vi "ViconIMUSimulation.vi"() -> ()   [LabVIEW 2016]
uses:
  DataProcess/CAlex2-Data/CAlex2_Data.lvclass
  D:/JinXin/LabVIEW.git/CAlex2-Controller-treadmill/Sim&Process/DataProcess/ExpData/ExpData.lvclass
  Classes/CAlex2-Display/CAlex2_Display.lvclass
  D:/JinXin/LabVIEW.git/CAlex2-Controller-treadmill/Classes/SerialChain/SerialChain.lvclass
  Classes/CAlex2/CAlex2.lvclass
  DataProcess/ExpData/ExpData.lvclass
  Classes/SerialChain/SerialChain.lvclass
panel:
  in  "New":refnum<k7>(container)
  in  "Old":refnum<k7>(container)
  in  "Path":path
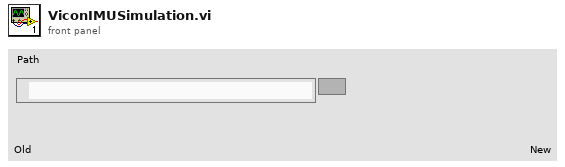
[diagram p1: front panel]
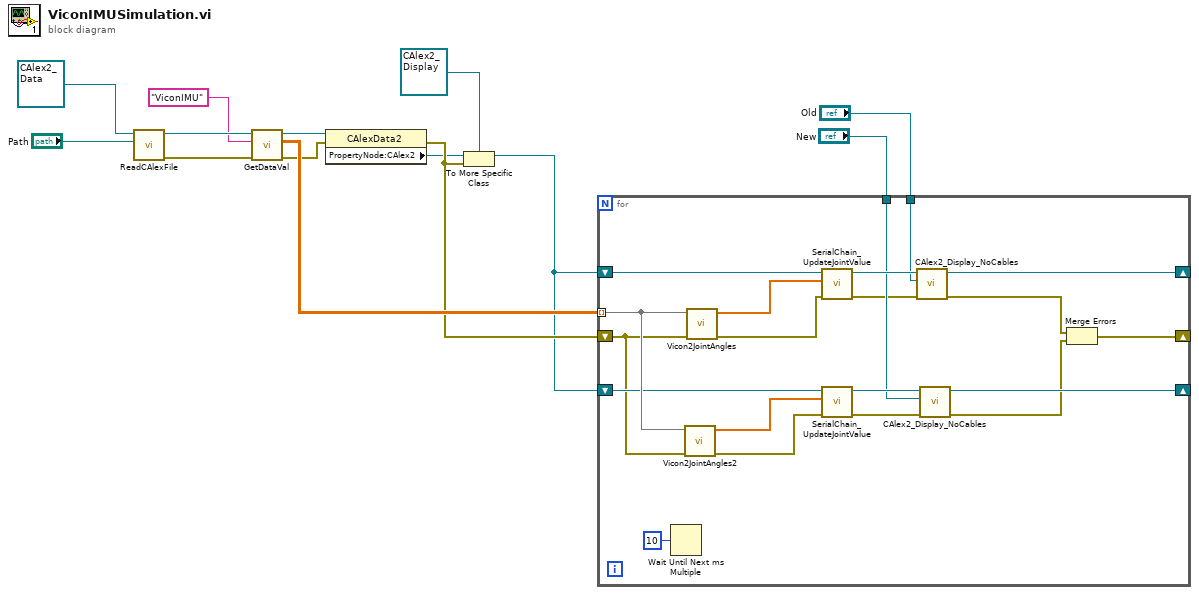
[diagram p0: block diagram]
diagram:
  n1 = call "ReadCAlexFile.vi"("ExpData File Path"="Path", "CAlexData2"=refnum<class "CAlex2_Data.lvclass"> refnum) -> ("error out"=w11:errorcluster, "CAlexData 2"=w12:refnum<class "CAlex2_Data.lvclass">)  [unwired: 8 in]
  n2 = call "GetDataVal.vi"("error in (no error)"=w11, "Name"="ViconIMU", "ExpData in"=w12) -> ("error out"=w7:errorcluster, "Data"=w9:dbl[][], "ExpData out"=w8:refnum<class "CAlex2_Data.lvclass">)  [unwired: 5 in, 1 out]
  n3 = property class="CAlexData2"(reference=w8, error in=w7) -> (error out=w6:errorcluster, "PropertyNode:CAlex2"=w5:refnum<class "CAlex2.lvclass">)  [unwired: 1 out]
  n4 = To More Specific Class(target class=refnum<class "CAlex2_Display.lvclass"> refnum ("CAlex2_Display.lvclass"), reference=w5, error in=w6) -> (specific class reference=w4:refnum<class "CAlex2_Display.lvclass">)  [unwired: 1 out]
  n5 = for {
    tunnel: w9 -> [w34] mode=indexing
    shift-right: [w18] -> _
    shift-left: w6 -> [w16]
    shift-right: [w25] -> _
    shift-left: w4 -> [w33]
    shift-right: [w28] -> _
    shift-left: w4 -> [w31]
    tunnel: "Old" -> [w24]
    tunnel: "New" -> [w23]
    n6 = Wait Until Next ms Multiple(millisecond multiple=u32 10) -> ()  [unwired: 1 out]
    n7 = call "Vicon2JointAngles2.vi"("error in (no error)"=w16, "ViconIMU in (rad)"=w34) -> ("error out"=w17:errorcluster, "Joint Angles (rad)"=w30:dbl[])  [unwired: 8 in]
    n8 = call "Vicon2JointAngles.vi"("error in (no error)"=w16, "ViconIMU in (rad)"=w34) -> ("error out"=w15:errorcluster, "Joint Angles (rad)"=w32:dbl[])  [unwired: 8 in]
    n9 = call "SerialChain_UpdateJointValue.vi"("error in (no error)"=w15, "JointAngle (rad | m)"=w32, "SerialChain in"=w33) -> ("error out"=w22:errorcluster, "SerialChain out"=w26:refnum<class "CAlex2_Display.lvclass">)  [unwired: 7 in]
    n10 = call "SerialChain_UpdateJointValue.vi"("error in (no error)"=w17, "JointAngle (rad | m)"=w30, "SerialChain in"=w31) -> ("error out"=w21:errorcluster, "SerialChain out"=w29:refnum<class "CAlex2_Display.lvclass">)  [unwired: 7 in]
    n11 = call "CAlex2_Display_NoCables.vi"("error in (no error)"=w22, "3D graph in"=w24, "CLX2 in"=w26) -> ("error out"=w19:errorcluster, "CLX2 out"=w25:refnum<class "CAlex2_Display.lvclass">)  [unwired: 5 in, 2 out]
    n12 = call "CAlex2_Display_NoCables.vi"("error in (no error)"=w21, "3D graph in"=w23, "CLX2 in"=w29) -> ("error out"=w20:errorcluster, "CLX2 out"=w28:refnum<class "CAlex2_Display.lvclass">)  [unwired: 5 in, 2 out]
    n13 = Merge Errors(w19, w20) -> (w18:errorcluster)
  }
